vi "MBtcp-WriteAny.vi"(0 "IP Address":string caption="IP Address(:Port(502)) (from Port Name)", 2 "Slave ID":u8=255 format="%.0x", 3 "Ch Name":string, 5 "Register":i32 caption="Register (from Ch.)", 7 "DataType(:RegisterType)":string, 9 "Value to Output":dbl, 11 "Error In":errorcluster) -> (15 "error out":errorcluster)   [LabVIEW 2020]
uses:
  RegisterTypes.ctl
panel:
  out "RegisterType":T1="Input" caption="RegisterType (from Comments)"
  out "Data type":string(combo) caption="Data type (from Comments)"
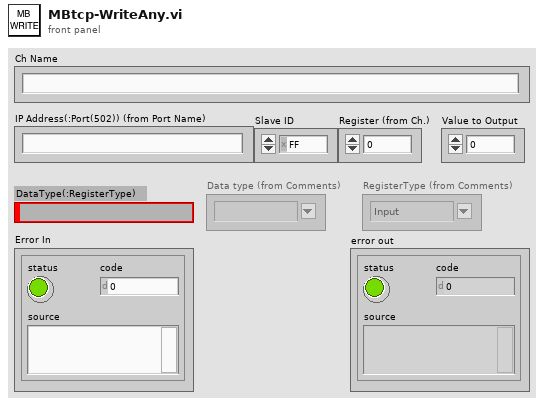
[diagram p1: front panel]
types:
  T1 = typedef "RegisterTypes.ctl" = string
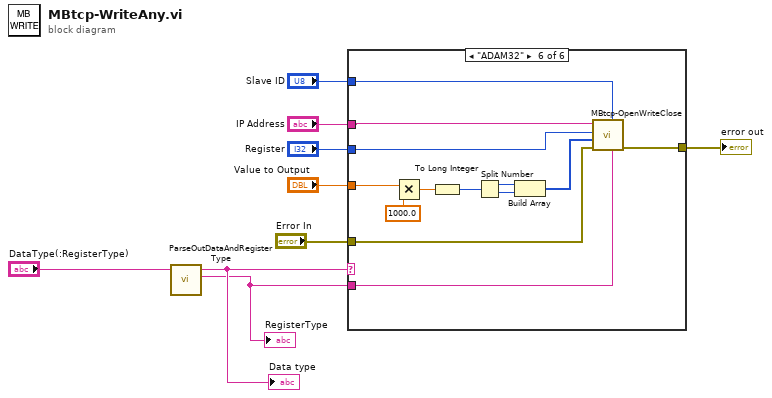
[diagram p0: block diagram]
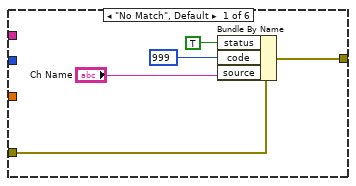
[diagram p2: hidden frame]
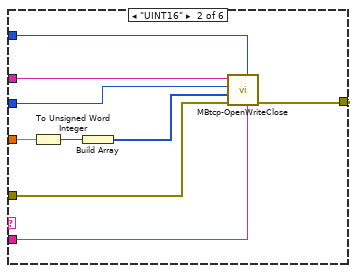
[diagram p3: hidden frame]
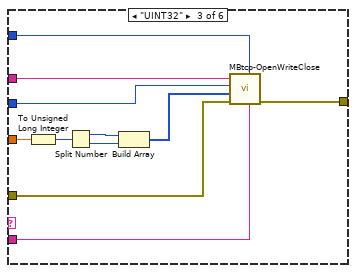
[diagram p4: hidden frame]
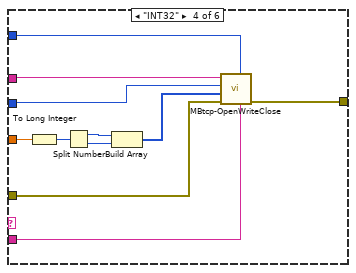
[diagram p5: hidden frame]
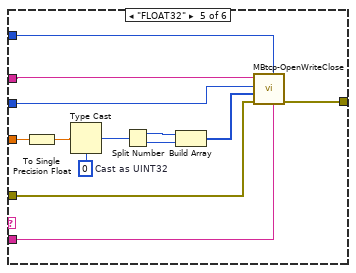
[diagram p6: hidden frame]
diagram:
  n1 = call "ParseOutDataAndRegisterType.vi"("DataType(:RegisterType) in"="DataType(:RegisterType)") -> ("RegisterType"=w2:string, "DataType"=w3:string)  [unwired: 9 in]
  "Data type" <- w3
  "RegisterType" <- w2
  n2 = case shown="\"ADAM32\"" w3 {
    tunnel: "IP Address" -> [_ w21 w30 w40 w51 w70]
    tunnel: "Register" -> [_ w20 w29 w39 w50 w69]
    tunnel: [w14 w18 w27 w41 w52 w71] -> w6
    tunnel: "Value to Output" -> [_ w23 w34 w44 w58 w64]
    tunnel: "Error In" -> [w10 w17 w26 w37 w48 w67]
    tunnel: "Slave ID" -> [_ w16 w25 w36 w47 w66]
    tunnel: w2 -> [_ w15 w24 w35 w46 w65]
    frame "No Match", Default {
      n3 = Bundle By Name(cluster=w10, "status"=TRUE, "code"=999, "source"="Ch Name") -> (w14:errorcluster)
    }
    frame "UINT16" {
      n4 = To Unsigned Word Integer(number=w23) -> (unsigned 16bit integer=w22:u16)
      n5 = Build Array(w22) -> (w19:u16[])
      n6 = call "MBtcp-OpenWriteClose.vi"("RegisterType"=w15, "Slave ID"=w16, "error in (no error)"=w17, "Values"=w19, "RegisterAddr"=w20, "IP Address(:port)"=w21) -> ("error out"=w18:errorcluster)  [unwired: 5 in]
    }
    frame "UINT32" {
      n7 = To Unsigned Long Integer(number=w34) -> (unsigned 32bit integer=w33:u32)
      n8 = Split Number(x=w33) -> (hi(x)=w31:u16, lo(x)=w32:u16)
      n9 = Build Array(w31, w32) -> (w28:u16[])
      n10 = call "MBtcp-OpenWriteClose.vi"("RegisterType"=w24, "Slave ID"=w25, "error in (no error)"=w26, "Values"=w28, "RegisterAddr"=w29, "IP Address(:port)"=w30) -> ("error out"=w27:errorcluster)  [unwired: 5 in]
    }
    frame "INT32" {
      n11 = To Long Integer(number=w44) -> (32bit integer=w45:i32)
      n12 = Split Number(x=w45) -> (hi(x)=w42:u16, lo(x)=w43:u16)
      n13 = Build Array(w42, w43) -> (w38:u16[])
      n14 = call "MBtcp-OpenWriteClose.vi"("RegisterType"=w35, "Slave ID"=w36, "error in (no error)"=w37, "Values"=w38, "RegisterAddr"=w39, "IP Address(:port)"=w40) -> ("error out"=w41:errorcluster)  [unwired: 5 in]
    }
    frame "FLOAT32" {
      w53 = u32 0  # Cast as UINT32
      n15 = To Single Precision Float(number=w58) -> (single precision float=w57:sgl)
      n16 = Type Cast(type=w53, x=w57) -> (*(type *) &x=w54:u32)
      n17 = Split Number(x=w54) -> (hi(x)=w55:u16, lo(x)=w56:u16)
      n18 = Build Array(w55, w56) -> (w49:u16[])
      n19 = call "MBtcp-OpenWriteClose.vi"("RegisterType"=w46, "Slave ID"=w47, "error in (no error)"=w48, "Values"=w49, "RegisterAddr"=w50, "IP Address(:port)"=w51) -> ("error out"=w52:errorcluster)  [unwired: 5 in]
    }
    frame "ADAM32" {
      n20 = Multiply(x=w64, y=1000.0) -> (x*y=w62:dbl)
      n21 = To Long Integer(number=w62) -> (32bit integer=w61:i32)
      n22 = Split Number(x=w61) -> (hi(x)=w60:u16, lo(x)=w59:u16)
      n23 = Build Array(w60, w59) -> (w68:u16[])
      n24 = call "MBtcp-OpenWriteClose.vi"("RegisterType"=w65, "Slave ID"=w66, "error in (no error)"=w67, "Values"=w68, "RegisterAddr"=w69, "IP Address(:port)"=w70) -> ("error out"=w71:errorcluster)  [unwired: 5 in]
    }
  }
  "error out" <- w6
